vi "Update SLSC Switch Property.vi"(8 "error in (no error)":errorcluster, 9 "Value":string, 10 "SLSC Switch Property":T1, 11 "SLSC Custom Device Ref in":T2 format="%.0x") -> (0 "error out":errorcluster, 3 "SLSC Custom Device  Ref out":T2 format="%.0x")   [LabVIEW 2017, in "SLSC Switch Scripting.lvlib"]
uses:
  SLSC Switch Scripting.lvlib
  <vilib>/NI Veristand/Custom Device API/Custom Device Item Ref.ctl
  SLSC Property Enum.ctl
  SLSC Scripting Constants.vi
  <vilib>/NI Veristand/Custom Device API/Set Item Property (String).vi
  <vilib>/NI VeriStand/Custom Device API/Custom Device API.lvlib
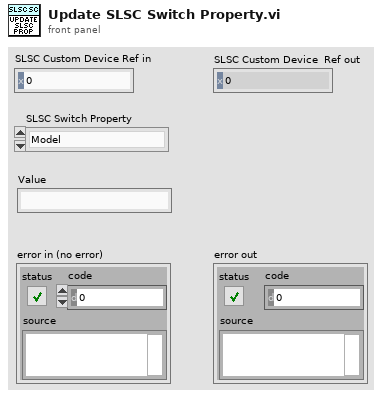
[diagram p1: front panel]
types:
  T1 = typedef "SLSC Switch Scripting.lvlib/SLSC Property Enum.ctl" = enum16{"Model", "Resource", "Topology", "Capabilities Version", "Capabilities"}
  T2 = typedef "Custom Device API.lvlib/Custom Device Item Ref.ctl" = u64
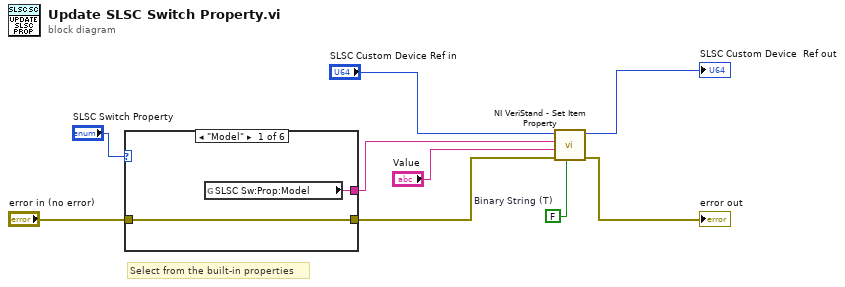
[diagram p0: block diagram]
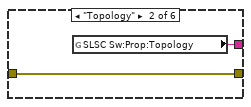
[diagram p2: hidden frame]
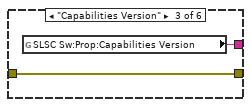
[diagram p3: hidden frame]
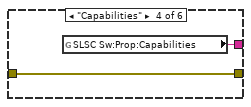
[diagram p4: hidden frame]
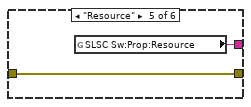
[diagram p5: hidden frame]
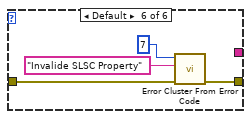
[diagram p6: hidden frame]
diagram:
  w5 = FALSE  # Binary String (T)
  # "Select from the built-in properties"
  n1 = case shown="\"Model\"" "SLSC Switch Property" {
    tunnel: [w11 w13 w15 w17 w19 _] -> w3
    tunnel: "error in (no error)" -> [w10 w12 w14 w16 w18 w21]
    tunnel: [w10 w12 w14 w16 w18 w20] -> w1
    frame "Model" {
      n2 = global read "SLSC Scripting Constants.vi" "SLSC Sw:Prop:Model"() -> (w11:string)
    }
    frame "Topology" {
      n3 = global read "SLSC Scripting Constants.vi" "SLSC Sw:Prop:Topology"() -> (w13:string)
    }
    frame "Capabilities Version" {
      n4 = global read "SLSC Scripting Constants.vi" "SLSC Sw:Prop:Capabilities Version"() -> (w15:string)
    }
    frame "Capabilities" {
      n5 = global read "SLSC Scripting Constants.vi" "SLSC Sw:Prop:Capabilities"() -> (w17:string)
    }
    frame "Resource" {
      n6 = global read "SLSC Scripting Constants.vi" "SLSC Sw:Prop:Resource"() -> (w19:string)
    }
    frame Default {
      n7 = call <vilib>:"Error Cluster From Error Code.vi"("error in (no error)"=w21, "error message (\"\")"="Invalide SLSC Property" ("error message (\"\")"), "error code (0)"=7) -> ("error out"=w20:errorcluster)  [unwired: 6 in]
    }
  }
  n8 = call-poly <vilib>:"NI VeriStand - Set Item Property.vi"("Binary String (T)"=w5, "error in (no error)"=w1, "Value"="Value", "Property Name"=w3, "Item Ref in"="SLSC Custom Device Ref in") -> ("error out"=→"error out":errorcluster, "Item Ref out"=→"SLSC Custom Device  Ref out":T2)  [unwired: 4 in, 1 out]
